vi "Check Collission.vi"(10 "Particle":refnum<class "Particle.lvclass">, 11 "Snake in":refnum<class "Snake.lvclass">) -> (2 "Collided?":bool, 3 "Snake out":refnum<class "Snake.lvclass">)   [LabVIEW 2020, in "Snake.lvclass"]
uses:
  Snake.lvclass
  Particle.lvclass
  Snake.lvclass/Snake.ctl
  Particle.lvclass/Particle.ctl
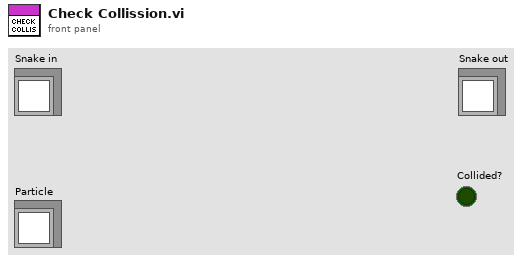
[diagram p1: front panel]
types:
  T1 = typedef "Particle.lvclass/Position.ctl" = cluster{"X":i32, "Y":i32}
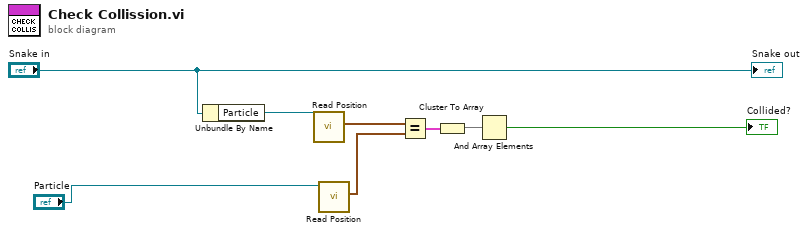
[diagram p0: block diagram]
diagram:
  n1 = Unbundle By Name("Snake in") -> ("Particle"=w7:refnum<class "Particle.lvclass">)
  n2 = call "Read Position.vi"("Particle in"=w7) -> ("Position"=w5:T1)  [unwired: 9 in, 1 out]
  n3 = call "Read Position.vi"("Particle in"="Particle") -> ("Position"=w4:T1)  [unwired: 9 in, 1 out]
  n4 = Equal?(x=w5, y=w4) -> (x = y?=w3:cluster{"X":bool, "Y":bool})
  n5 = Cluster To Array(cluster=w3) -> (array=w2:bool[])
  n6 = And Array Elements(Boolean array=w2) -> (logical AND=→"Collided?":bool)
  "Snake out" <- "Snake in"
